vi "DAQmx.Clear.vi"(8 "error in (no error)":errorcluster, 11 "DAQmx in":refnum<class "DAQmx.lvclass">) -> (0 "error out":errorcluster, 3 "DAQmx out":refnum<class "DAQmx.lvclass">)   [LabVIEW 2020, in "DAQmx.lvclass"]
uses:
  DAQmx.lvclass
  DAQmx.lvclass/DAQmx.ctl
  <userlib>/_OpenG.lib/time/time.llb/openg_time.lvlib
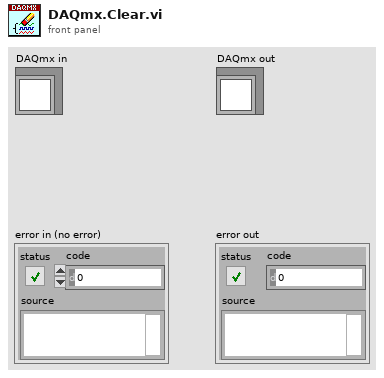
[diagram p1: front panel]
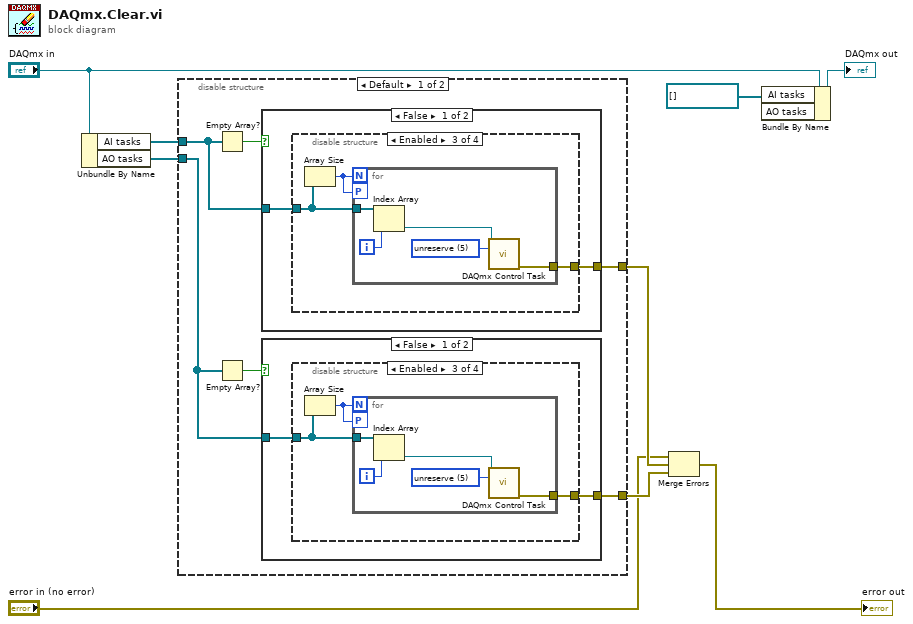
[diagram p0: block diagram]
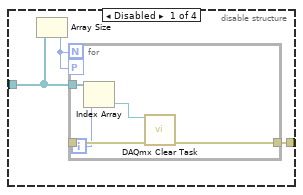
[diagram p2: hidden frame]
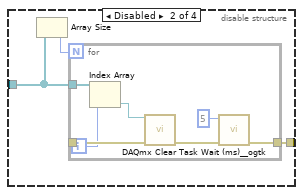
[diagram p3: hidden frame]
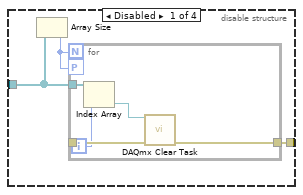
[diagram p6: hidden frame]
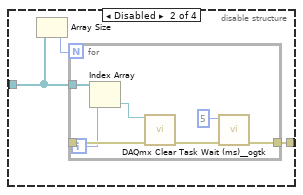
[diagram p7: hidden frame]
diagram:
  w5 = refnum<k21>[] [] ("AI task")
  n1 = Unbundle By Name("DAQmx in") -> ("AI tasks"=w8:refnum<k21>[], "AO tasks"=w9:refnum<k21>[])
  n2 = disable-structure shown="Default" {
    disable-tunnel: [w15 _] -> w3
    disable-tunnel: w9 -> [w12 _]
    disable-tunnel: w8 -> [w13 _]
    disable-tunnel: [w11 _] -> w4
    frame condition #0 (active) {
      n3 = Empty Array?(array=w13) -> (empty?=w14:bool)
      n4 = Empty Array?(array=w12) -> (empty?=w10:bool)
      n5 = case shown="False" w14 {
        tunnel: w13 -> [w46 _]
        tunnel: [w47 _] -> w15
        frame False {
          n6 = disable-structure shown="Enabled" {
            disable-tunnel: [w51 w60 w70 _] -> w47
            disable-tunnel: w46 -> [w48 w57 w69 _]
            frame Disabled {
              n7 = Array Size(array=w48) -> (size(s)=w49:i32)
              n8 = for {
                N: w49 -> [_]
                tunnel: w48 -> [w54]
                tunnel: [w56] -> w50
                tunnel: [w53] -> w51
                workers-P: w49 -> [_]
                i -> [w55]
                n9 = Index Array(array=w54, index=w55) -> (element=w52:refnum<k21>)
                n10 = call <vilib>:"DAQmx Clear Task.vi"("task in"=w52, "error in"=w56) -> ("error out"=w53:errorcluster)  [unwired: 13 in]
              }
            }
            frame Disabled {
              n11 = Array Size(array=w57) -> (size(s)=w58:i32)
              n12 = for {
                N: w58 -> [_]
                tunnel: w57 -> [w65]
                tunnel: [w67] -> w59
                tunnel: [w62] -> w60
                i -> [w66]
                n13 = Index Array(array=w65, index=w66) -> (element=w63:refnum<k21>)
                n14 = call <vilib>:"DAQmx Clear Task.vi"("task in"=w63, "error in"=w67) -> ("error out"=w64:errorcluster)  [unwired: 13 in]
                n15 = call <userlib>:"Wait (ms)__ogtk.vi"("error in (no error)"=w64, "milliseconds to wait"=u32 5) -> ("error out"=w62:errorcluster)  [unwired: 8 in, 1 out]
              }
            }
            frame Enabled {
              n16 = Array Size(array=w69) -> (size(s)=w68:i32)
              n17 = for {
                N: w68 -> [_]
                tunnel: w69 -> [w74]
                tunnel: [w71] -> w70
                workers-P: w68 -> [_]
                i -> [w75]
                w73 = 5 items=["verify"=2, "reserve"=4, "commit"=3, "unreserve"=5, "abort"=6] ("action")
                n18 = Index Array(array=w74, index=w75) -> (element=w72:refnum<k21>)
                n19 = call <vilib>:"DAQmx Control Task.vi"("task/channels in"=w72, "action"=w73) -> ("error out"=w71:errorcluster)  [unwired: 12 in, 1 out]
              }
            }
            frame Disabled {
            }
          }
        }
        frame True {
        }
      }
      n20 = case shown="False" w10 {
        tunnel: w12 -> [w16 _]
        tunnel: [w17 _] -> w11
        frame False {
          n21 = disable-structure shown="Enabled" {
            disable-tunnel: [w21 w30 w40 _] -> w17
            disable-tunnel: w16 -> [w18 w27 w39 _]
            frame Disabled {
              n22 = Array Size(array=w18) -> (size(s)=w19:i32)
              n23 = for {
                N: w19 -> [_]
                tunnel: w18 -> [w24]
                tunnel: [w26] -> w20
                tunnel: [w23] -> w21
                workers-P: w19 -> [_]
                i -> [w25]
                n24 = Index Array(array=w24, index=w25) -> (element=w22:refnum<k21>)
                n25 = call <vilib>:"DAQmx Clear Task.vi"("task in"=w22, "error in"=w26) -> ("error out"=w23:errorcluster)  [unwired: 13 in]
              }
            }
            frame Disabled {
              n26 = Array Size(array=w27) -> (size(s)=w28:i32)
              n27 = for {
                N: w28 -> [_]
                tunnel: w27 -> [w35]
                tunnel: [w37] -> w29
                tunnel: [w32] -> w30
                i -> [w36]
                n28 = Index Array(array=w35, index=w36) -> (element=w33:refnum<k21>)
                n29 = call <vilib>:"DAQmx Clear Task.vi"("task in"=w33, "error in"=w37) -> ("error out"=w34:errorcluster)  [unwired: 13 in]
                n30 = call <userlib>:"Wait (ms)__ogtk.vi"("error in (no error)"=w34, "milliseconds to wait"=u32 5) -> ("error out"=w32:errorcluster)  [unwired: 8 in, 1 out]
              }
            }
            frame Enabled {
              n31 = Array Size(array=w39) -> (size(s)=w38:i32)
              n32 = for {
                N: w38 -> [_]
                tunnel: w39 -> [w44]
                tunnel: [w41] -> w40
                workers-P: w38 -> [_]
                i -> [w45]
                w43 = 5 items=["verify"=2, "reserve"=4, "commit"=3, "unreserve"=5, "abort"=6] ("action")
                n33 = Index Array(array=w44, index=w45) -> (element=w42:refnum<k21>)
                n34 = call <vilib>:"DAQmx Control Task.vi"("task/channels in"=w42, "action"=w43) -> ("error out"=w41:errorcluster)  [unwired: 12 in, 1 out]
              }
            }
            frame Disabled {
            }
          }
        }
        frame True {
        }
      }
    }
    frame condition #1 {
    }
  }
  n35 = Merge Errors("error in (no error)", w3, w4) -> (→"error out":errorcluster)
  n36 = Bundle By Name(cluster="DAQmx in", "AI tasks"=w5, "AO tasks"=w5) -> (→"DAQmx out":refnum<class "DAQmx.lvclass">)
